vi "RUSHClimber.vi"(1 "In Cluster":T2) -> (0 "Out Cluster":T3)   [LabVIEW 2012]
panel:
  in  "Rot Lowest POT pos":dbl=2.4
  in  "Rot Highest POT pot":dbl=2.6
  in  "Ext Highest POT pos":dbl
  in  "Ext Lowest POT pos":dbl
  out "ClimbConst":T1
  out "ClimbPOTDep":dbl
  out "ClimbManualDep":dbl
  out "ClimbManualExt":dbl
  in  "Extension Speed":dbl=0.75
  in  "Deploy Speed":dbl=0.75
  in  "Deadband":dbl=0.1
  # "For Local use only"
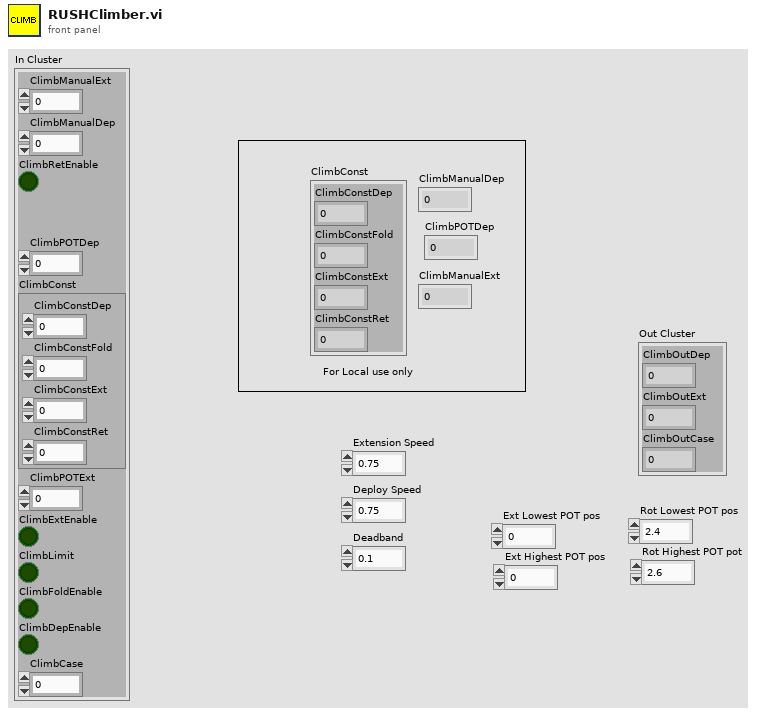
[diagram p1: front panel]
types:
  T1 = cluster{"ClimbConstDep":dbl, "ClimbConstFold":dbl, "ClimbConstExt":dbl, "ClimbConstRet":dbl}
  T2 = cluster{"ClimbManualExt":dbl, "ClimbManualDep":dbl, "ClimbRetEnable":bool, "ClimbPOTDep":dbl, "ClimbConst":cluster{"ClimbConstDep":dbl, "ClimbConstFold":dbl, "ClimbConstExt":dbl, "ClimbConstRet":dbl}, "ClimbPOTExt":dbl, "ClimbExtEnable":bool, "ClimbLimit":bool, "ClimbFoldEnable":bool, "ClimbDepEnable":bool, "ClimbCase":dbl}
  T3 = cluster{"ClimbOutDep":dbl, "ClimbOutExt":dbl, "ClimbOutCase":i32}
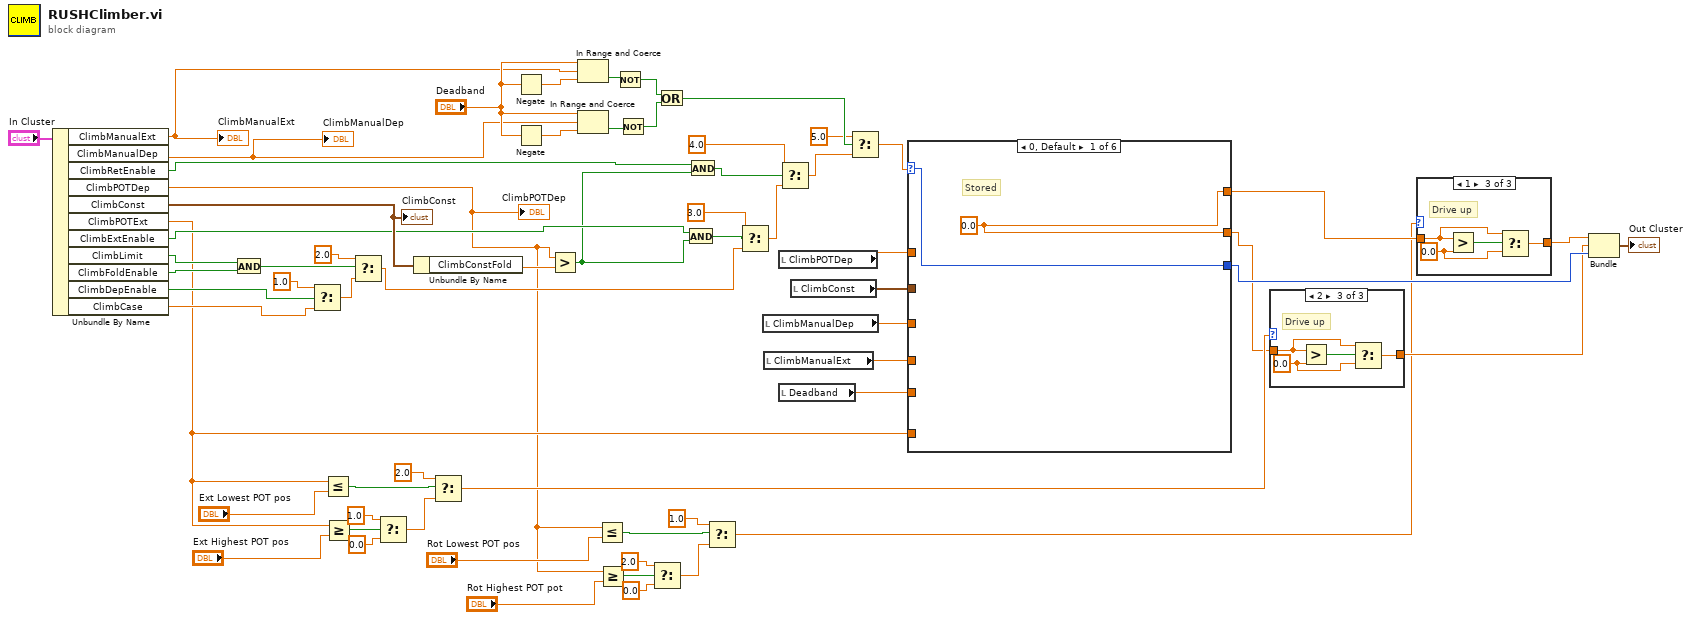
[diagram p0: block diagram]
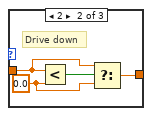
[diagram p3: hidden frame]
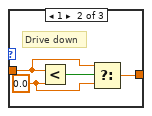
[diagram p5: hidden frame]
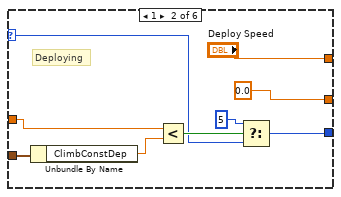
[diagram p6: hidden frame]
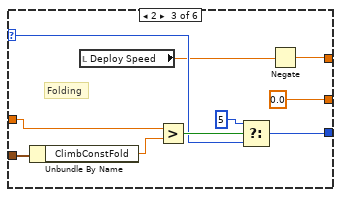
[diagram p7: hidden frame]
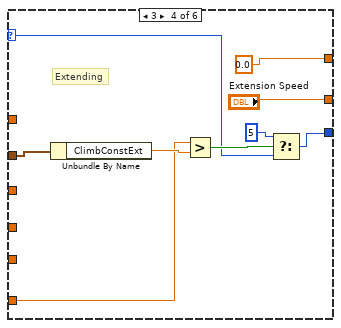
[diagram p8: hidden frame]
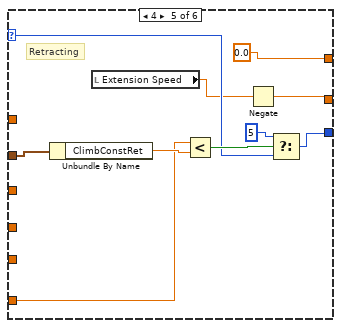
[diagram p9: hidden frame]
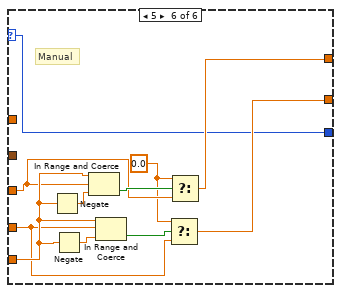
[diagram p10: hidden frame]
diagram:
  n1 = Unbundle By Name("In Cluster") -> ("ClimbManualExt"=w37:dbl, "ClimbManualDep"=w36:dbl, "ClimbRetEnable"=w35:bool, "ClimbPOTDep"=w4:dbl, "ClimbConst"=w34:T1, "ClimbPOTExt"=w16:dbl, "ClimbExtEnable"=w33:bool, "ClimbLimit"=w32:bool, "ClimbFoldEnable"=w31:bool, "ClimbDepEnable"=w28:bool, "ClimbCase"=w30:dbl)
  "ClimbManualExt" <- w37
  "ClimbManualDep" <- w36
  "ClimbPOTDep" <- w4
  "ClimbConst" <- w34
  n2 = And(x=w32, y=w31) -> (x .and. y?=w62:bool)
  n3 = Select(t=1.0, s=w28, f=w30) -> (s? t:f=w61:dbl)
  n4 = Less Or Equal?(x=w16, y="Ext Lowest POT pos") -> (x <= y?=w18:bool)
  n5 = Greater Or Equal?(x=w16, y="Ext Highest POT pos") -> (x >= y?=w22:bool)
  n6 = Select(t=2.0, s=w62, f=w61) -> (s? t:f=w53:dbl)
  n7 = Select(t=1.0, s=w22, f=0.0) -> (s? t:f=w19:dbl)
  n8 = Unbundle By Name(w34) -> ("ClimbConstFold"=w50:dbl)
  n9 = Select(t=2.0, s=w18, f=w19) -> (s? t:f=w15:dbl)
  n10 = Negate(x="Deadband") -> (-x=w63:dbl)
  n11 = Negate(x="Deadband") -> (-x=w64:dbl)
  n12 = Greater?(x=w4, y=w50) -> (0:w25:bool)
  n13 = In Range and Coerce(upper limit="Deadband", x=w37, lower limit=w63) -> (In Range?=w46:bool)  [unwired: 1 out]
  n14 = In Range and Coerce(upper limit="Deadband", x=w36, lower limit=w64) -> (In Range?=w47:bool)  [unwired: 1 out]
  n15 = Less Or Equal?(x=w4, y="Rot Lowest POT pos") -> (x <= y?=w11:bool)
  n16 = Greater Or Equal?(x=w4, y="Rot Highest POT pot") -> (x >= y?=w7:bool)
  n17 = Not(x=w46) -> (.not. x?=w45:bool)
  n18 = Not(x=w47) -> (.not. x?=w44:bool)
  n19 = Select(t=2.0, s=w7, f=0.0) -> (s? t:f=w10:dbl)
  n20 = Or(x=w45, y=w44) -> (x .or. y?=w43:bool)
  n21 = And(x=w33, y=w25) -> (x .and. y?=w59:bool)
  n22 = And(x=w35, y=w25) -> (x .and. y?=w55:bool)
  n23 = Select(t=1.0, s=w11, f=w10) -> (s? t:f=w1:dbl)
  n24 = Select(t=3.0, s=w59, f=w53) -> (s? t:f=w57:dbl)
  n25 = local read "ClimbManualDep"() -> (w48:dbl)
  n26 = local read "ClimbManualExt"() -> (w42:dbl)
  n27 = local read "ClimbPOTDep"() -> (w51:dbl)
  n28 = local read "Deadband"() -> (w41:dbl)
  n29 = Select(t=4.0, s=w55, f=w57) -> (s? t:f=w27:dbl)
  n30 = local read "ClimbConst"() -> (w49:T1)
  n31 = Select(t=5.0 ("f"), s=w43, f=w27) -> (s? t:f=w52:dbl)
  n32 = case shown="0, Default" w52 {
    selector: w52 -> [w65 w71 w81 w91 w101 w105]
    tunnel: w51 -> [_ w73 w83 _ _ _]
    tunnel: w49 -> [_ w75 w85 w90 w100 _]
    tunnel: [w65 w69 w79 w88 w98 w105] -> w40
    tunnel: [w66 "Deploy Speed" w76 0.0 ("Extend Speed") 0.0 ("Extend Speed") w107] -> w3
    tunnel: [w66 0.0 ("Extend Speed") 0.0 ("Extend Speed") "Extension Speed" w95 w106] -> w14
    tunnel: w48 -> [_ _ _ _ _ w110]
    tunnel: w42 -> [_ _ _ _ _ w108]
    tunnel: w41 -> [_ _ _ _ _ w113]
    tunnel: w16 -> [_ _ _ w89 w99 _]
    frame 0, Default {
      w66 = 0.0
      # "Stored"
    }
    frame 1 {
      # "Deploying"
      n33 = Unbundle By Name(w75) -> ("ClimbConstDep"=w74:dbl)
      n34 = Less?(x=w73, y=w74) -> (x < y?=w72:bool)
      n35 = Select(t=5, s=w72, f=w71) -> (s? t:f=w69:i32)
    }
    frame 2 {
      # "Folding"
      n36 = Unbundle By Name(w85) -> ("ClimbConstFold"=w84:dbl)
      n37 = local read "Deploy Speed"() -> (w77:dbl)
      n38 = Greater?(x=w83, y=w84) -> (0:w82:bool)
      n39 = Select(t=5, s=w82, f=w81) -> (s? t:f=w79:i32)
      n40 = Negate(x=w77) -> (-x=w76:dbl)
    }
    frame 3 {
      # "Extending"
      n41 = Unbundle By Name(w90) -> ("ClimbConstExt"=w94:dbl)
      n42 = Greater?(x=w89, y=w94) -> (0:w93:bool)
      n43 = Select(t=5, s=w93, f=w91) -> (s? t:f=w88:i32)
    }
    frame 4 {
      # "Retracting"
      n44 = Unbundle By Name(w100) -> ("ClimbConstRet"=w104:dbl)
      n45 = local read "Extension Speed"() -> (w96:dbl)
      n46 = Less?(x=w99, y=w104) -> (x < y?=w103:bool)
      n47 = Negate(x=w96) -> (-x=w95:dbl)
      n48 = Select(t=5, s=w103, f=w101) -> (s? t:f=w98:i32)
    }
    frame 5 {
      w109 = 0.0 ("t")
      # "Manual"
      n49 = Negate(x=w113) -> (-x=w114:dbl)
      n50 = Negate(x=w113) -> (-x=w115:dbl)
      n51 = In Range and Coerce(upper limit=w113, x=w110, lower limit=w114) -> (In Range?=w111:bool)  [unwired: 1 out]
      n52 = In Range and Coerce(upper limit=w113, x=w108, lower limit=w115) -> (In Range?=w112:bool)  [unwired: 1 out]
      n53 = Select(t=w109, s=w112, f=w108) -> (s? t:f=w106:dbl)
      n54 = Select(t=w109, s=w111, f=w110) -> (s? t:f=w107:dbl)
    }
  }
  n55 = case shown="2" w15 {
    tunnel: w14 -> [w116 w118 w122]
    tunnel: [w116 w117 w121] -> w13
    frame 0, Default {
      # "All good"
    }
    frame 1 {
      w119 = 0.0 ("y")
      # "Drive down"
      n56 = Less?(x=w118, y=w119) -> (x < y?=w120:bool)
      n57 = Select(t=w118, s=w120, f=w119) -> (s? t:f=w117:dbl)
    }
    frame 2 {
      w123 = 0.0 ("y")
      # "Drive up"
      n58 = Greater?(x=w122, y=w123) -> (0:w124:bool)
      n59 = Select(t=w122, s=w124, f=w123) -> (s? t:f=w121:dbl)
    }
  }
  n60 = case shown="1" w1 {
    tunnel: w3 -> [w125 w127 w131]
    tunnel: [w125 w126 w130] -> w2
    frame 0, Default {
      # "All good"
    }
    frame 2 {
      w128 = 0.0 ("y")
      # "Drive down"
      n61 = Less?(x=w127, y=w128) -> (x < y?=w129:bool)
      n62 = Select(t=w127, s=w129, f=w128) -> (s? t:f=w126:dbl)
    }
    frame 1 {
      w132 = 0.0 ("y")
      # "Drive up"
      n63 = Greater?(x=w131, y=w132) -> (0:w133:bool)
      n64 = Select(t=w131, s=w133, f=w132) -> (s? t:f=w130:dbl)
    }
  }
  n65 = Bundle("y"=w2, "y"=w13, "t"=w40) -> (→"Out Cluster":cluster{"y":dbl, "y":dbl, "t":i32})  [unwired: 1 in]
